vi "Add State(s) to Queue By BOOL(Array All).vi"(4 "FALSE (\"\")":string[](array[string]), 6 "TRUE (\"\")":string[](array[string]), 8 "High Priority? (F)":bool, 10 "Condition":bool, 11 "State Queue (\"\")":string) -> (3 "Remaining States":string)   [LabVIEW 2017, in "Communicable State Machine.lvlib"]
doc: "Generates the concatenated state of TRUE/FALSE and the remaining states based on the <b>High Priority</b> and Boolean inputs. The <b>High Priority</b> input determines whether to concatenate the TRUE or FALSE string before or after the remaining states. The <b>TRUE</b> and <b>FALSE</b> inputs determine whether the string to be concatenated is TRUE or FALSE.\n\n\n> [!NOTE] <b>CSM State Queue Operation API</b>\n>\n> This type of API only concatenates message strings and does not send messages directly. The message is sent and the operation executed within the Parse State Queue++ VI. Unlike the Message Building API, this type of API includes a CSM state queue string input, which is equivalent to inserting a message into the state queue.\n\n\n-- <b>Controls</b> --\n- <b>State Queue (\"\")</b>: The entire state queue is connected to this input.\n- <b>Condition</b>: Selects the state string connected to the TRUE or FALSE terminal.\n- <b>High Priority? (F)</b>: If TRUE, the state is inserted at the front of the <b>State Queue (\"\")</b>. If FALSE, the state is appended to the end.\n- <b>TRUE (\"\")</b>: The state string to insert when <b>Condition</b> is TRUE.\n- <b>FALSE (\"\")</b>: The state string to insert when <b>Condition</b> is FALSE.\n\n-- <b>Indicators</b> --\n- <b>Remaining States</b>: Returns all concatenated states and arguments."
uses:
  Communicable State Machine.lvlib
  _Shared/CSM Shared.lvlib
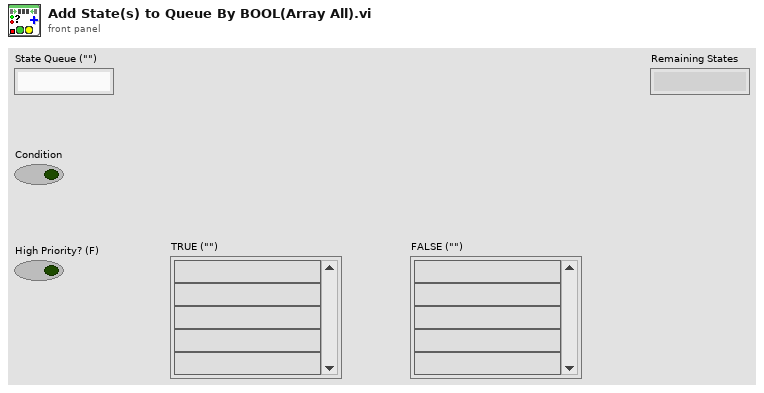
[diagram p1: front panel]
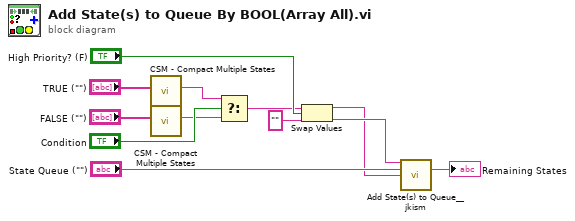
[diagram p0: block diagram]
diagram:
  n1 = call "CSM - Compact Multiple States.vi"("Multiple States"="TRUE (\"\")") -> ("States"=w2:string)  [unwired: 9 in]
  n2 = call "CSM - Compact Multiple States.vi"("Multiple States"="FALSE (\"\")") -> ("States"=w1:string)  [unwired: 9 in]
  n3 = Select(t=w2, s="Condition", f=w1) -> (s? t:f=w6:string)
  n4 = Swap Values(12:w6, 13:"High Priority? (F)", 14:"") -> (1:w3:string, 3:w4:string)
  n5 = call "Add State(s) to Queue__jkism.vi"("State(s) in Front (\"\")"=w4, "State(s) in (\"\")"="State Queue (\"\")", "State(s) at Back (\"\")"=w3) -> ("States Out"=→"Remaining States":string)  [unwired: 12 in]
